vi "SetValueString.vi"(7 "LabVIEW Web Service Request":refnum<class "Web Request.lvclass">, 11 "ControlName":string) -> (1 "Error":i32, 2 "ErrorString":string, 3 "dataOut":string)   [LabVIEW 2024]
uses:
  <vilib>/wsapi/Web Request.lvclass
  g_VIServerPort.vi
panel:
  in  "ControlValue":string
  out "value":string
  out "errorOut":errorcluster
  # "Use the Web Service Request input terminal to call the VIs on the Web Services palette. Do not remove it from the connector pane unless you don't need access to the palette."
  # "Each additional control wired to the connector pane will be available as an input in the URL. To include an indicator in terminal-mode output (the default setting), it must also be wired to the connector pane."
  # "http://127.0.0.1:8001/WebService/SetValueNumeric?ControlName={value}"
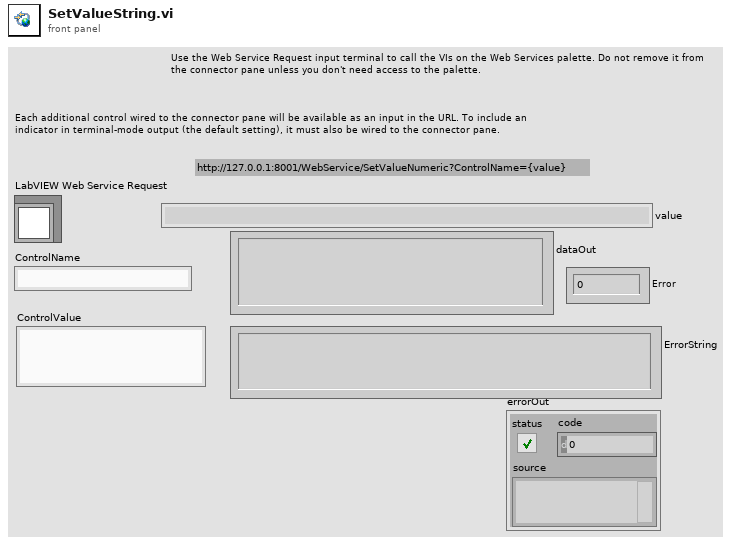
[diagram p1: front panel]
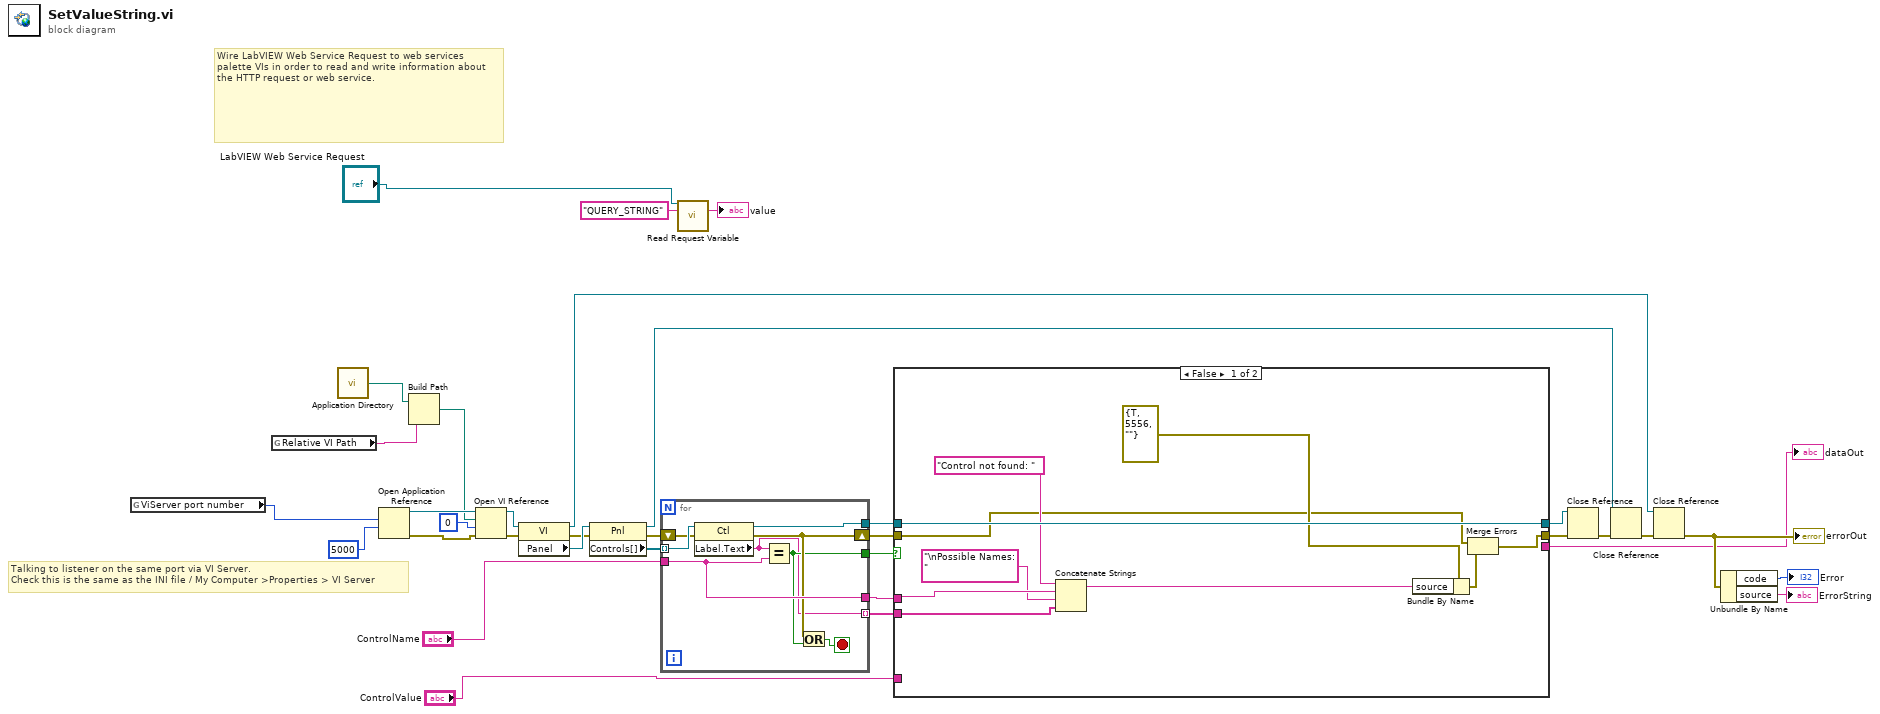
[diagram p0: block diagram]
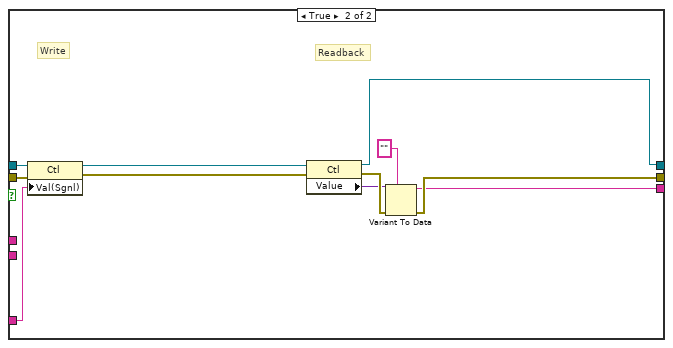
[diagram p2: hidden frame]
diagram:
  # "Talking to listener on the same port via VI Server.\nCheck this is the same as the INI file / My Computer >Properties > VI Server"
  # "Wire LabVIEW Web Service Request to web services palette VIs in order to read and write information about the HTTP request or web service."
  n1 = global read "g_VIServerPort.vi" "ViServer port number"() -> (w4:u16)
  n2 = global read "g_VIServerPort.vi" "Relative VI Path"() -> (w1:string)
  n3 = call <vilib>:"Application Directory.vi"() -> ("Application Directory"=w9:path)
  n4 = Open Application Reference(9:5000 ("timeout ms (60000)"), 10:w4) -> (0:w15:errorcluster, 3:w16:refnum<vi>)  [unwired: 2 in]
  n5 = Build Path(base path=w9, name or relative path=w1) -> (appended path=w8:path)
  n6 = Open VI Reference(application reference (local)=w16, vi path=w8, options=0, error in (no error)=w15) -> (vi reference=w18:refnum<vi>, error out=w30:errorcluster)  [unwired: 2 in]
  n7 = property class="VI"(reference=w18, error in=w30) -> (reference out=w25:refnum<vi>, error out=w29:errorcluster, "Panel"=w33:refnum<vi>)
  n8 = property class="Pnl"(reference=w33, error in=w29) -> (reference out=w19:refnum<vi>, error out=w28:errorcluster, "Controls[]"=w32:refnum<vi>[])
  n9 = for {
    tunnel: w32 -> [w42] mode=indexing
    tunnel: "ControlName" -> [w39]
    tunnel: [w36] -> w27
    tunnel: [w40] -> w20
    tunnel: [w39] -> w17
    shift-right: [w37] -> w21
    shift-left: w28 -> [w41]
    tunnel: [w35] -> w11 mode=indexing
    stop <- w38 stop-if-true
    n10 = property class="Ctl"(reference=w42, error in=w41) -> (reference out=w40:refnum<vi>, error out=w37:errorcluster, "Label.Text"=w35:string)
    n11 = Equal?(x=w35, y=w39) -> (x = y?=w36:bool)
    n12 = Or(x=w37, y=w36) -> (x .or. y?=w38:bool)
  }
  n13 = call <vilib>:"Read Request Variable.vi"("LabVIEW Web Service Request"="LabVIEW Web Service Request", "variable name"="QUERY_STRING") -> ("value"=→"value":string)  [unwired: 11 in, 2 out]
  n14 = case shown="False" w27 {
    tunnel: w20 -> [w52 w63]
    tunnel: [w52 w60] -> w26
    tunnel: [w46 w54] -> w22
    tunnel: w21 -> [w47 w62]
    tunnel: w17 -> [w45 _]
    tunnel: w11 -> [w43 _]
    tunnel: "ControlValue" -> [_ w59]
    tunnel: [_ w53] -> w2
    frame False {
      n15 = Concatenate Strings("Control not found: " ("string"), w45, "\nPossible Names: " ("string"), w43) -> (w50:string)
      n16 = Bundle By Name(cluster=errorcluster {"status"=TRUE, "code"=5556, "source"=""} ("error constant"), "source"=w50) -> (w48:errorcluster)
      n17 = Merge Errors(w47, w48) -> (w46:errorcluster)
    }
    frame True {
      # "Readback"
      # "Write"
      n18 = property class="Ctl"(reference=w63, error in=w62, "Val(Sgnl)"=w59) -> (reference out=w57:refnum<vi>, error out=w56:errorcluster)
      n19 = property class="Ctl"(reference=w57, error in=w56) -> (reference out=w60:refnum<vi>, error out=w61:errorcluster, "Value"=w58:variant)
      n20 = Variant To Data(error in=w61, type="", Variant=w58) -> (data=w53:string, error out=w54:errorcluster)
    }
  }
  "dataOut" <- w2
  n21 = Close Reference(reference=w26, error in (no error)=w22) -> (error out=w24:errorcluster)
  n22 = Close Reference(reference=w19, error in (no error)=w24) -> (error out=w23:errorcluster)
  n23 = Close Reference(reference=w25, error in (no error)=w23) -> (error out=w14:errorcluster)
  "errorOut" <- w14
  n24 = Unbundle By Name(w14) -> ("code"=→"Error":i32, "source"=→"ErrorString":string)
